vi "AngleToElbowEncoder.vi"(11 "angle(deg)":dbl) -> (3 "encoderPulses":i32)   [LabVIEW 2018]
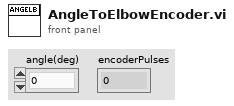
[diagram p1: front panel]
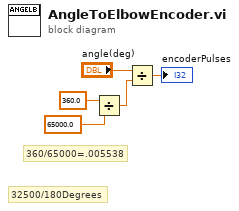
[diagram p0: block diagram]
diagram:
  # "360/65000=.005538"
  # "32500/180Degrees"
  n1 = Divide(x=360.0, y=65000.0) -> (x/y=w2:dbl)
  n2 = Divide(x="angle(deg)", y=w2) -> (x/y=→"encoderPulses":dbl)
